vi "Create Pattern Script(OpCode).vi"(8 "error in (no error)":errorcluster, 10 "Write Script in":string, 11 "BML Pattern Creater in":refnum<class "BML Pattern Creater.lvclass">) -> (0 "error out":errorcluster, 2 "Script out":string, 3 "BML Pattern Creater out":refnum<class "BML Pattern Creater.lvclass">)   [LabVIEW 2018, in "BML Pattern Creater.lvlib" / "BML Pattern Creater.lvclass"]
uses:
  BML Pattern Creater.lvclass
  C:/P4 Workspace/PC Client/Solutions/5g_eap/trunk/1.0/HiSi5GmmWave/Pattern_Gen_Tool/Interfaces/Protocol Interface.lvlibp/Interfaces/Protocol Interface/Protocol Interface.lvclass
  BML Pattern Creater.lvclass/BML Pattern Creater.ctl
  Interfaces/Protocol Interface.lvlibp/Interfaces/Protocol Interface/Pin State.ctl
  Special Frame.ctl
  Interfaces/Protocol Interface.lvlibp/Interfaces/Protocol Interface/Read Period(ms).vi
  Interfaces/Protocol Interface.lvlibp/Interfaces/Protocol Interface/Protocol Interface.lvclass
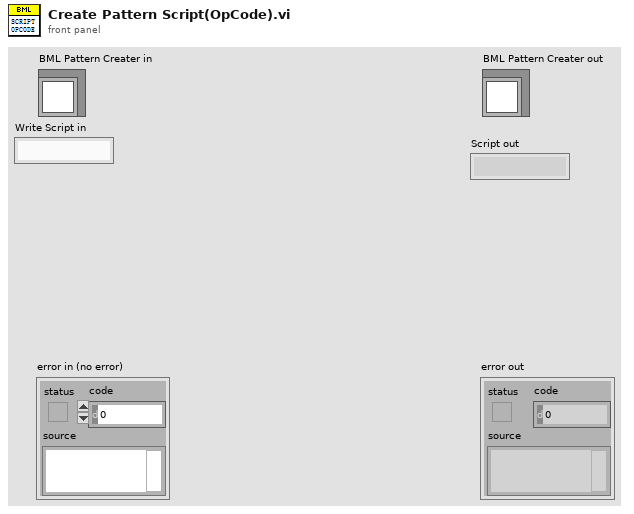
[diagram p1: front panel]
types:
  T1 = typedef "BML Pattern Creater.lvlib/BML Pattern Creater.lvclass/Special Frame.ctl" = enum16{"Sync Header", "BML Header", "SW Trig", "SetID State", "Exit SetID State", "SW Reset", "Wait"}
  T2 = typedef "Protocol Interface.lvlibp/Protocol Interface.lvclass/Pin State.ctl" = enum16{"0", "1", "L", "H", "X", "V", "D", "M"}
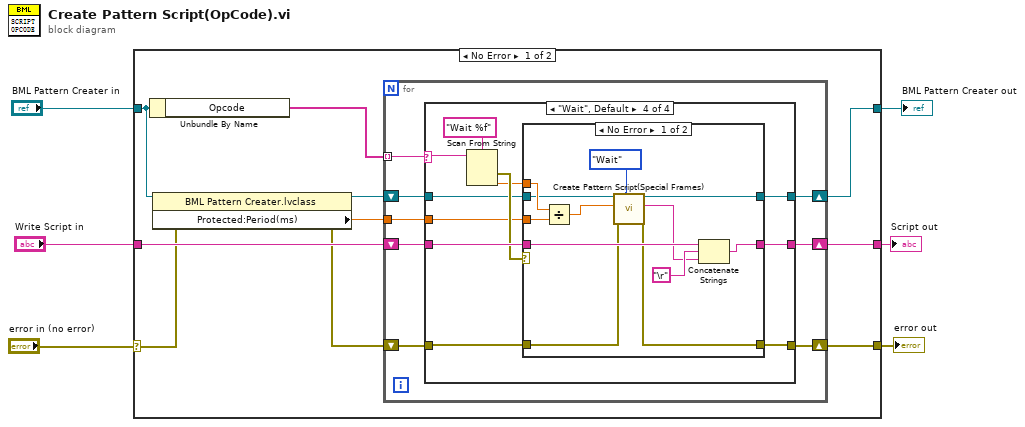
[diagram p0: block diagram]
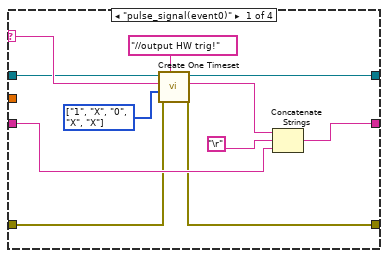
[diagram p2: hidden frame]
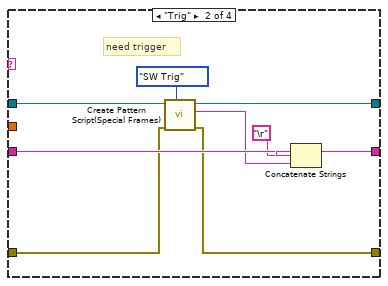
[diagram p3: hidden frame]
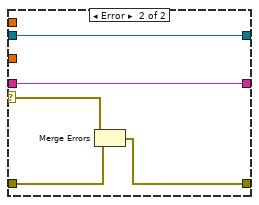
[diagram p5: hidden frame]
diagram:
  n1 = case shown="No Error" "error in (no error)" {
    selector: "error in (no error)" -> [w10 w77]
    tunnel: [w13 w77] -> w5
    tunnel: [w14 w76] -> w3
    tunnel: "BML Pattern Creater in" -> [w12 w76]
    tunnel: "Write Script in" -> [w15 _]
    tunnel: [w7 _] -> w1
    frame No Error {
      n2 = Unbundle By Name(w12) -> ("Opcode"=w16:string[])
      n3 = property class="BML Pattern Creater.lvclass"(reference=w12, error in=w10) -> (reference out=w9:refnum<class "BML Pattern Creater.lvclass">, error out=w11:errorcluster, "Protected:Period(ms)"=w8:dbl)
      n4 = for {
        shift-right: [w21] -> w7
        shift-left: w15 -> [w24]
        shift-right: [w22] -> w13
        shift-left: w11 -> [w23]
        tunnel: w16 -> [w20] mode=indexing
        shift-right: [w18] -> w14
        shift-left: w9 -> [w19]
        tunnel: w8 -> [w17]
        n5 = case shown="\"Wait\", Default" w20 {
          selector: w20 -> [w29 _ _ w55]
          tunnel: w24 -> [w34 w43 w47 w57]
          tunnel: w23 -> [w25 w40 w46 w53]
          tunnel: [w33 w44 w47 w58] -> w21
          tunnel: [w27 w39 w46 w56] -> w22
          tunnel: w19 -> [w28 w37 w45 w50]
          tunnel: [w26 w36 w45 w48] -> w18
          tunnel: w17 -> [_ _ _ w49]
          frame "pulse_signal(event0)" {
            w30 = T2[] [enum."1", enum."X", enum."0", enum."X", enum."X"] items=["0", "1", "L", "H", "X", "V", "D", "M"] ("Pin State")
            n6 = call-dynamic "Create One Timeset.vi"("Notes"="//output HW trig!", "error in (no error)"=w25, "Pin State"=w30, "opcode"=w29, "BML Pattern Creater in"=w28) -> ("error out"=w27:errorcluster, "string out"=w32:string, "BML Pattern Creater out"=w26:refnum<class "BML Pattern Creater.lvclass">)  [unwired: 4 in]
            n7 = Concatenate Strings(w32, "\r", w34) -> (w33:string)
          }
          frame "Trig" {
            # "need trigger"
            n8 = call "Create Pattern Script(Special Frames).vi"("Special Frame Type"=Special_Frame."SW Trig", "error in (no error)"=w40, "BML Pattern Creater in"=w37) -> ("error out"=w39:errorcluster, "string out"=w38:string, "BML Pattern Creater out"=w36:refnum<class "BML Pattern Creater.lvclass">)  [unwired: 6 in]
            n9 = Concatenate Strings(w43, "\r", w38) -> (w44:string)
          }
          frame "" {
          }
          frame "Wait", Default {
            n10 = Scan From String(format string="Wait %f", input string=w55) -> (error out=w52:errorcluster, output 1=w51:dbl)  [unwired: 3 in, 2 out]
            n11 = case shown="No Error" w52 {
              selector: w52 -> [_ w74]
              tunnel: [w70 w75] -> w58
              tunnel: w57 -> [w69 w75]
              tunnel: [w66 w72] -> w56
              tunnel: w51 -> [w64 _]
              tunnel: w53 -> [w67 w73]
              tunnel: w50 -> [w60 w71]
              tunnel: w49 -> [w63 _]
              tunnel: [w59 w71] -> w48
              frame No Error {
                n12 = Divide(x=w64, y=w63) -> (x/y=w62:dbl)
                n13 = call "Create Pattern Script(Special Frames).vi"("Special Frame Type"=Special_Frame."Wait", "error in (no error)"=w67, "Num of Timeset"=w62, "BML Pattern Creater in"=w60) -> ("error out"=w66:errorcluster, "string out"=w61:string, "BML Pattern Creater out"=w59:refnum<class "BML Pattern Creater.lvclass">)  [unwired: 5 in]
                n14 = Concatenate Strings(w69, "\r", w61) -> (w70:string)
              }
              frame Error {
                n15 = Merge Errors(w74, w73) -> (w72:errorcluster)
              }
            }
          }
        }
      }
    }
    frame Error {
    }
  }
  "error out" <- w5
  "BML Pattern Creater out" <- w3
  "Script out" <- w1
